vi "przalaczanie kanalow na osi Y.vi"() -> ()   [LabVIEW 2013]
uses:
  <vilib>/measure/NI_MABase.lvlib
panel:
  out "Mixed Signal Graph":waveform(dbl)[](graph)
  out "Waveform Graph":waveform(dbl)[](graph)
  in  "Ustawienia":T1(array[cluster])=[{"signal type"=enum."Sine Wave", "frequency"=5.0, "amplitude"=79.95673866091062, "phase"=0.0}, {"signal type"=enum."Sine Wave", "frequency"=5.0, "amplitude"=627.7475412679432, "phase"=0.0}, {"signal type"=enum."Sine Wave", "frequency"=5.0, "amplitude"=8.922382456517203, "phase"=0.0}, {"signal type"=enum."Sine Wave", "frequency"=5.0, "amplitude"=8.22107792428465, "phase"=0.0}, {"signal type"=enum."Sine Wave", "frequency"=5.0, "amplitude"=1.0, "phase"=0.0}] {"phase" format="%.2p"; "amplitude" format="%0.2p"; "frequency" format="%#_13g"}
  in  "sampling info":cluster{"Fs":dbl, "#s":dbl}={"Fs"=200.0, "#s"=100.0} {"Fs" format="%.2p"}
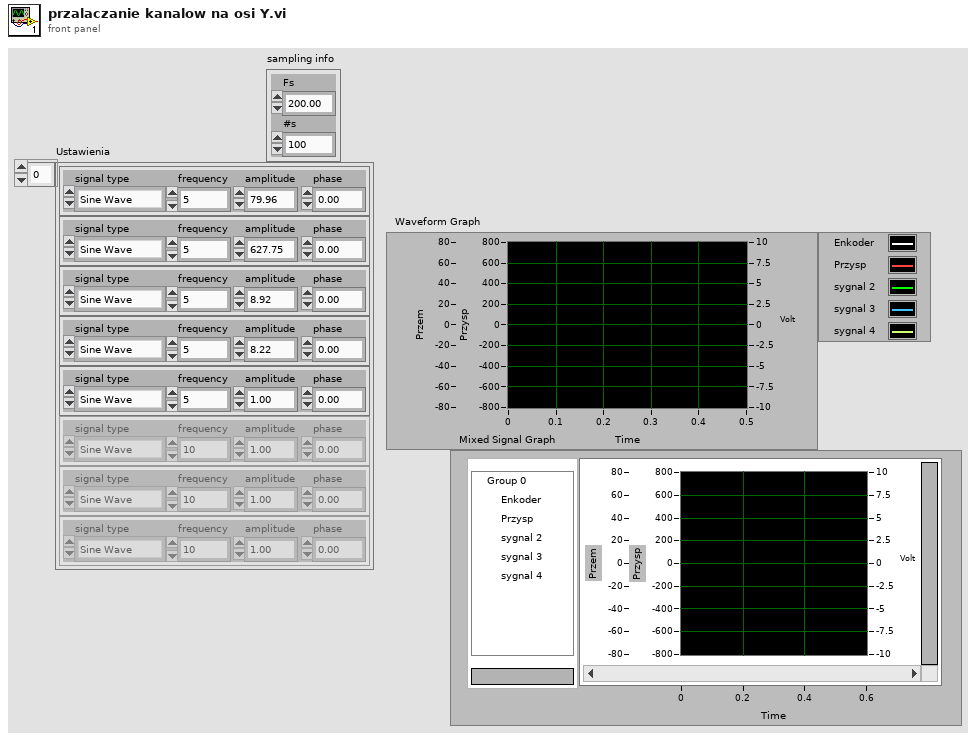
[diagram p1: front panel]
types:
  T1 = cluster{"signal type":enum16{"Sine Wave", "Triangle Wave", "Square Wave", "Sawtooth Wave"}, "frequency":dbl, "amplitude":dbl, "phase":dbl}[]
  T2 = cluster{"signal type":enum16{"Sine Wave", "Triangle Wave", "Square Wave", "Sawtooth Wave"}, "frequency":dbl, "amplitude":dbl, "phase":dbl}
  T3 = enum16{"Sine Wave", "Triangle Wave", "Square Wave", "Sawtooth Wave"}
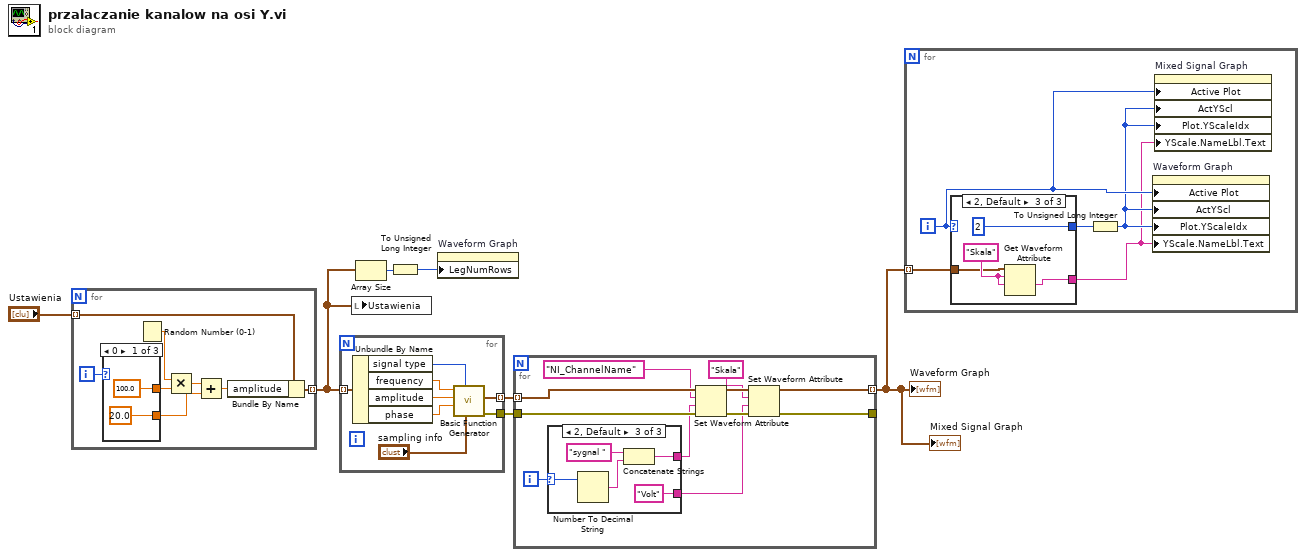
[diagram p0: block diagram]
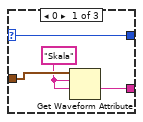
[diagram p2: hidden frame]
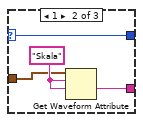
[diagram p3: hidden frame]
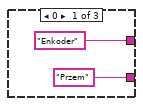
[diagram p4: hidden frame]
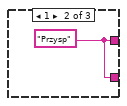
[diagram p5: hidden frame]
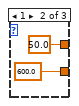
[diagram p6: hidden frame]
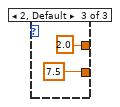
[diagram p7: hidden frame]
diagram:
  n1 = for {
    tunnel: "Ustawienia" -> [w15] mode=indexing
    tunnel: [w14] -> w4 mode=indexing
    i -> [w13]
    n2 = case shown="0" w13 {
      tunnel: [100.0 ("y") 50.0 ("y") 2.0 ("y")] -> w11
      tunnel: [20.0 ("y") 600.0 ("y") 7.5 ("y")] -> w9
      frame 0 {
      }
      frame 1 {
      }
      frame 2, Default {
      }
    }
    n3 = Random Number (0-1)() -> (number: 0 to 1=w12:dbl)
    n4 = Multiply(x=w12, y=w11) -> (x*y=w10:dbl)
    n5 = Add(x=w10, y=w9) -> (x+y=w8:dbl)
    n6 = Bundle By Name(cluster=w15, "amplitude"=w8) -> (w14:T2)
  }
  n7 = for {
    tunnel: w4 -> [w28] mode=indexing
    tunnel: [w23] -> w6 mode=indexing
    tunnel: [w22] -> w5
    n8 = Unbundle By Name(w28) -> ("signal type"=w27:T3, "frequency"=w26:dbl, "amplitude"=w25:dbl, "phase"=w24:dbl)
    n9 = call <vilib>:"Basic Function Generator.vi"("sampling info"="sampling info", "signal type"=w27, "phase"=w24, "amplitude"=w25, "frequency"=w26) -> ("error out"=w22:errorcluster, "signal out"=w23:waveform(dbl))  [unwired: 4 in, 1 out]
  }
  n10 = local write "Ustawienia"(w4) -> ()
  n11 = Array Size(array=w4) -> (size(s)=w3:i32)
  n12 = To Unsigned Long Integer(number=w3) -> (unsigned 32bit integer=w2:u32)
  n13 = property on="Waveform Graph" class="WFGraph (strict)"("LegNumRows"=w2) -> ()  [unwired: 2 in, 2 out]
  n14 = for {
    tunnel: w6 -> [w39] mode=indexing
    tunnel: w5 -> [w40]
    tunnel: [w32] -> w1 mode=indexing
    tunnel: [w33] -> _
    i -> [w37]
    n15 = case shown="2, Default" w37 {
      selector: w37 -> [_ _ w45]
      tunnel: ["Enkoder" ("name") w43 w46] -> w36
      tunnel: ["Przem" ("name") w43 "Volt" ("name")] -> w30
      frame 0 {
      }
      frame 1 {
        w43 = "Przysp" ("name")
      }
      frame 2, Default {
        n16 = Number To Decimal String(number=w45) -> (decimal integer string=w47:string)  [unwired: 1 in]
        n17 = Concatenate Strings("sygnal " ("name"), w47) -> (w46:string)
      }
    }
    n18 = Set Waveform Attribute(4:w40, 5:w36, 6:"NI_ChannelName" ("name"), 7:w39) -> (0:w35:errorcluster, 3:w34:waveform(dbl))  [unwired: 1 out]
    n19 = Set Waveform Attribute(4:w35, 5:w30, 6:"Skala" ("name"), 7:w34) -> (0:w33:errorcluster, 3:w32:waveform(dbl))  [unwired: 1 out]
  }
  "Waveform Graph" <- w1
  "Mixed Signal Graph" <- w1
  n20 = for {
    tunnel: w1 -> [w52] mode=indexing
    i -> [w51]
    n21 = case shown="2, Default" w51 {
      selector: w51 -> [w57 w61 _]
      tunnel: [w57 w61 2] -> w53
      tunnel: w52 -> [w56 w59 w63]
      tunnel: [w54 w58 w62] -> w49
      frame 0 {
        w55 = "Skala" ("name")
        n22 = Get Waveform Attribute(5:w55, 6:w55, 7:w56) -> (1:w54:string)  [unwired: 1 in, 3 out]
      }
      frame 1 {
        w60 = "Skala" ("name")
        n23 = Get Waveform Attribute(5:w60, 6:w60, 7:w59) -> (1:w58:string)  [unwired: 1 in, 3 out]
      }
      frame 2, Default {
        w64 = "Skala" ("name")
        n24 = Get Waveform Attribute(5:w64, 6:w64, 7:w63) -> (1:w62:string)  [unwired: 1 in, 3 out]
      }
    }
    n25 = To Unsigned Long Integer(number=w53) -> (unsigned 32bit integer=w50:u32)
    n26 = property on="Waveform Graph" class="WFGraph (strict)"("Active Plot"=w51, "ActYScl"=w50, "Plot.YScaleIdx"=w50, "YScale.NameLbl.Text"=w49) -> ()  [unwired: 2 in, 2 out]
    n27 = property on="Mixed Signal Graph" class="MixedGraph (strict)"("Active Plot"=w51, "ActYScl"=w50, "Plot.YScaleIdx"=w50, "YScale.NameLbl.Text"=w49) -> ()  [unwired: 2 in, 2 out]
  }
